vi "Create Function String (Efficiency).vi"(8 "error in (no error)":errorcluster, 10 "Function (1: Eta1)":i32(ring)=1 items=["Eta1"=1, "Eta2"=2, "Eta3"=3, "Eta4"=4], 11 "VISA resource name":refnum<visa-resource-name>) -> (0 "error out":errorcluster, 2 "Function String":string, 3 "VISA resource name out":refnum<visa-resource-name>)   [LabVIEW 2021, in "Yokogawa WT1800 Series.lvlib"]
doc: "Create a efficiency function string"
uses:
  <instrlib>/Yokogawa WT1800 Series/Yokogawa WT1800 Series.lvlib
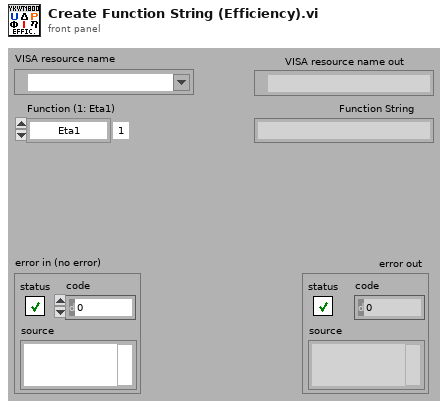
[diagram p1: front panel]
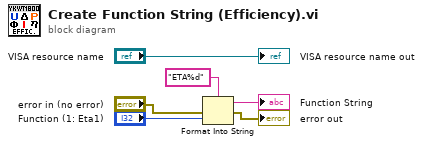
[diagram p0: block diagram]
diagram:
  n1 = Format Into String(format string="ETA%d" ("形式文字列"), error in="error in (no error)", "Function (1: Eta1)") -> (resulting string=→"Function String":string, error out=→"error out":errorcluster)  [unwired: 1 in]
  "VISA resource name out" <- "VISA resource name"
